vi "Get Scale Labels.vi"(11 "波形数组":waveform(dbl)[](array[waveform])) -> (1 "Y标尺标签文本":string, 2 "X标尺标签文本":string)   [LabVIEW 2022 SP3]
doc: "返回波形数组中第一个波形的标尺标签。 如波形属性中未设定标尺，则返回“时间”和“幅值”分别作为X标签和Y标签。"
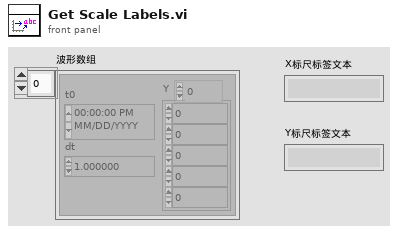
[diagram p1: front panel]
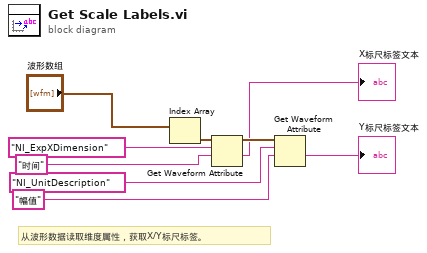
[diagram p0: block diagram]
diagram:
  # "从波形数据读取维度属性，获取X/Y标尺标签。"
  n1 = Index Array(array="波形数组") -> (element=w2:waveform(dbl))  [unwired: 1 in]
  n2 = Get Waveform Attribute(5:"时间" ("Time"), 6:"NI_ExpXDimension", 7:w2) -> (1:→"X标尺标签文本":string, 3:w5:waveform(dbl))  [unwired: 1 in, 2 out]
  n3 = Get Waveform Attribute(5:"幅值" ("Amplitude"), 6:"NI_UnitDescription", 7:w5) -> (1:→"Y标尺标签文本":string)  [unwired: 1 in, 3 out]
